vi "Zadanie 2 v. 2.0..vi"() -> ()   [LabVIEW 2020]
panel:
  out "# elements in queue":i32
  out "Obecnie generowana liczba":dbl
  out "Liczby":dbl[](array[numeric])
  out "Zajêtoœæ":bool
  in  "stop":bool
  out "Zliczenie producent":i32
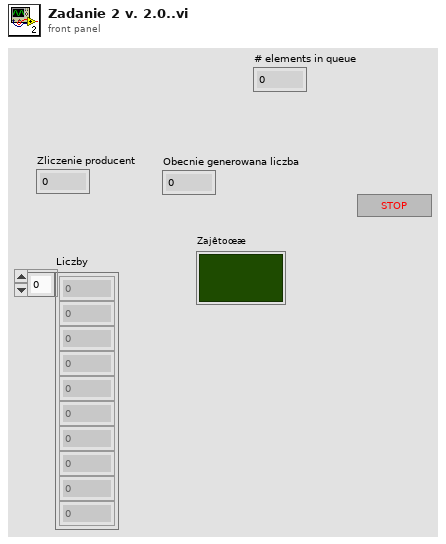
[diagram p1: front panel]
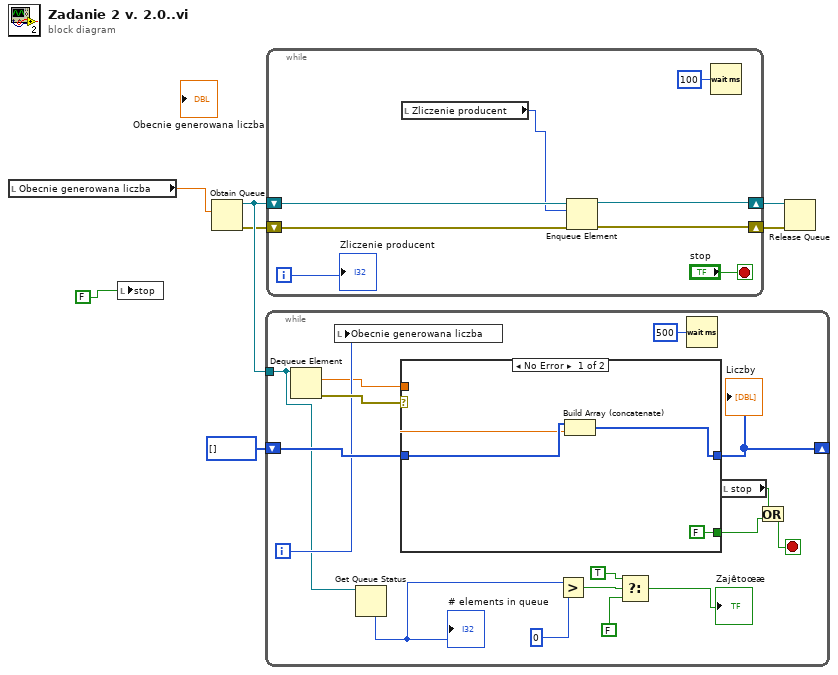
[diagram p0: block diagram]
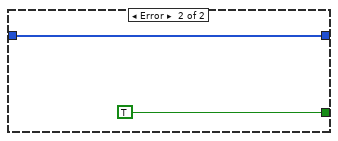
[diagram p2: hidden frame]
diagram:
  n1 = local read "Obecnie generowana liczba"() -> (w3:dbl)
  n2 = local write "stop"(FALSE) -> ()
  n3 = Obtain Queue(element data type=w3) -> (queue out=w7:refnum<queue>, error out=w6:errorcluster)  [unwired: 4 in, 1 out]
  n4 = while {
    tunnel: w7 -> [w17]
    shift-right: [w21] -> _
    shift-left: i32[] [] -> [w22]
    i -> [w19]
    stop <- w10 stop-if-true
    n5 = Dequeue Element(queue=w17) -> (element=w18:dbl, error out=w23:errorcluster)  [unwired: 2 in, 2 out]
    n6 = local write "Obecnie generowana liczba"(w19) -> ()
    n7 = Get Queue Status(queue=w17) -> (# elements in queue=w16:i32)  [unwired: 2 in, 7 out]
    "# elements in queue" <- w16
    n8 = case shown="No Error" w23 {
      tunnel: w18 -> [w25 _]
      tunnel: [FALSE TRUE] -> w9
      tunnel: [w27 w28] -> w21
      tunnel: w22 -> [w26 w28]
      frame No Error {
        n9 = Build Array (concatenate)(w26, w25) -> (w27:i32[])
      }
      frame Error {
      }
    }
    "Liczby" <- w21
    n10 = Greater?(x=w16, y=0) -> (0:w14:bool)
    n11 = Select(t=TRUE, s=w14, f=FALSE) -> (s? t:f=→"Zajêtoœæ":bool)
    n12 = Wait (ms)(milliseconds to wait=u32 500) -> ()  [unwired: 1 out]
    n13 = local read "stop"() -> (w8:bool)
    n14 = Or(x=w8, y=w9) -> (x .or. y?=w10:bool)
  }
  n15 = while {
    shift-right: [w33] -> w4
    shift-left: w6 -> [w34]
    shift-right: [w35] -> w5
    shift-left: w7 -> [w36]
    i -> [w31]
    stop <- "stop" stop-if-true
    n16 = local read "Zliczenie producent"() -> (w30:i32)
    n17 = Enqueue Element(queue=w36, element=w30, error in (no error)=w34) -> (queue out=w35:refnum<queue>, error out=w33:errorcluster)  [unwired: 1 in, 1 out]
    n18 = Wait (ms)(milliseconds to wait=u32 100) -> ()  [unwired: 1 out]
    "Zliczenie producent" <- w31
  }
  n19 = Release Queue(queue=w5, error in (no error)=w4) -> ()  [unwired: 1 in, 3 out]
